vi "Bring Up lvBeacons.vi"(8 "Error In":errorcluster) -> (0 "Error Out":errorcluster)   [LabVIEW 2013]
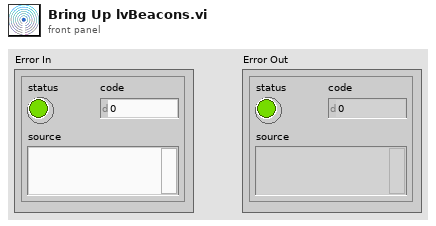
[diagram p1: front panel]
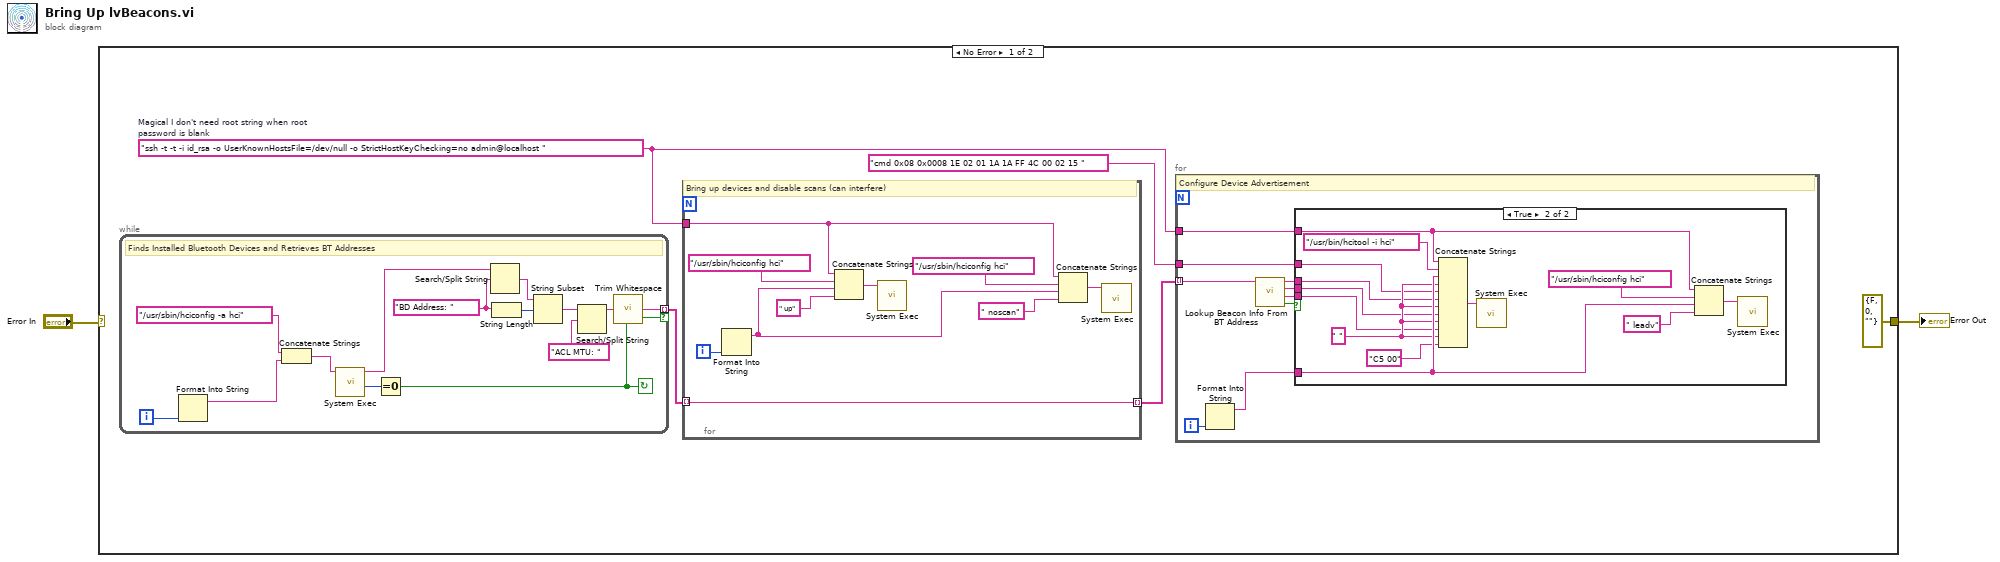
[diagram p0: block diagram]
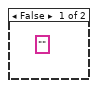
[diagram p2: hidden frame]
diagram:
  n1 = case shown="No Error" "Error In" {
    selector: "Error In" -> [_ w54]
    tunnel: [errorcluster {"status"=FALSE, "code"=0, "source"=""} ("error IO") w54] -> w1
    frame No Error {
      w5 = "ssh -t -t -i id_rsa -o UserKnownHostsFile=/dev/null -o StrictHostKeyChecking=no admin@localhost "  # Magical I don't need root string when root password is blank
      n2 = while {
        tunnel: [w46] -> w7 mode=indexing if=w44
        i -> [w41]
        stop <- w44 continue-if-true
        w50 = "BD Address: " ("search string/char (-)")
        # "Finds Installed Bluetooth Devices and Retrieves BT Addresses"
        n3 = Format Into String(w41) -> (resulting string=w40:string)  [unwired: 3 in, 1 out]
        n4 = Concatenate Strings("/usr/sbin/hciconfig -a hci" ("command line"), w40) -> (w42:string)
        n5 = call <vilib>:"System Exec.vi"("command line"=w42) -> ("return code"=w45:i32, "standard output"=w47:string)  [unwired: 7 in, 2 out]
        n6 = Equal To 0?(x=w45) -> (x = 0?=w44:bool)
        n7 = Search/Split String(string=w47, search string/char (-)=w50) -> (match + rest of string=w49:string)  [unwired: 1 in, 2 out]
        n8 = String Length(string=w50) -> (length=w52:i32)
        n9 = String Subset(string=w49, offset (0)=w52) -> (substring=w51:string)  [unwired: 1 in]
        n10 = Search/Split String(string=w51, search string/char (-)="ACL MTU: ") -> (substring before match=w53:string)  [unwired: 1 in, 2 out]
        n11 = call <vilib>:"Trim Whitespace.vi"("string"=w53) -> ("trimmed string"=w46:string)  [unwired: 1 in]
      }
      n12 = for {
        tunnel: w7 -> [w30] mode=indexing
        tunnel: w5 -> [w31]
        tunnel: [w30] -> w6 mode=indexing
        i -> [w38]
        # "Bring up devices and disable scans (can interfere)"
        n13 = Format Into String(w38) -> (resulting string=w32:string)  [unwired: 3 in, 1 out]
        n14 = Concatenate Strings(w31, "/usr/sbin/hciconfig hci" ("command line"), w32, " up" ("string")) -> (w36:string)
        n15 = call <vilib>:"System Exec.vi"("command line"=w36) -> ()  [unwired: 7 in, 4 out]
        n16 = Concatenate Strings(w31, "/usr/sbin/hciconfig hci" ("command line"), w32, " noscan" ("string")) -> (w35:string)
        n17 = call <vilib>:"System Exec.vi"("command line"=w35) -> ()  [unwired: 7 in, 4 out]
      }
      n18 = for {
        tunnel: w6 -> [w16] mode=indexing
        tunnel: w5 -> [w11]
        tunnel: "cmd 0x08 0x0008 1E 02 01 1A 1A FF 4C 00 02 15 " ("command line") -> [w10]
        i -> [w9]
        # "Configure Device Advertisement"
        n19 = Format Into String(w9) -> (resulting string=w8:string)  [unwired: 3 in, 1 out]
        n20 = call "Lookup Beacon Info From BT Address.vi"("BT Address"=w16) -> ("found?"=w15:bool, "Minor"=w14:string, "Major"=w13:string, "UUID"=w12:string)  [unwired: 7 in]
        n21 = case shown="True" w15 {
          tunnel: w14 -> [_ w24]
          tunnel: w13 -> [_ w25]
          tunnel: w12 -> [_ w26]
          tunnel: w11 -> [_ w17]
          tunnel: w10 -> [_ w27]
          tunnel: w8 -> [_ w29]
          frame False {
            (unwired) ""
          }
          frame True {
            w28 = " "
            n22 = Concatenate Strings(w17, "/usr/bin/hcitool -i hci", w29, w28, w27, w26, w28, w25, w28, w24, w28, "C5 00" ("string")) -> (w21:string)
            n23 = call <vilib>:"System Exec.vi"("command line"=w21) -> ()  [unwired: 7 in, 4 out]
            n24 = Concatenate Strings(w17, "/usr/sbin/hciconfig hci" ("command line"), w29, " leadv" ("string")) -> (w18:string)
            n25 = call <vilib>:"System Exec.vi"("command line"=w18) -> ()  [unwired: 7 in, 4 out]
          }
        }
      }
    }
    frame Error {
    }
  }
  "Error Out" <- w1
